vi "Write Maximum Channel Length.vi"(8 "error in (no error)":errorcluster, 10 "maximum data length":i32, 11 "Data in":refnum<class "Data.lvclass">) -> (0 "error out":errorcluster, 3 "Data out":refnum<class "Data.lvclass">)   [LabVIEW 2017, in "Data.lvclass"]
uses:
  <vilib>/addons/_NISVFA/_Shared subVIs/Data Objects/Data/Data.lvclass
  <vilib>/addons/_NISVFA/_Shared subVIs/Data Objects/Data/Data.lvclass/Data.ctl
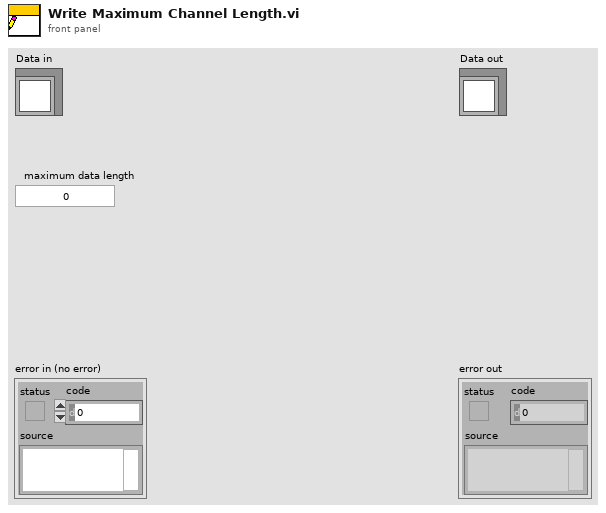
[diagram p1: front panel]
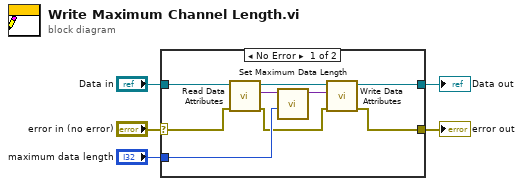
[diagram p0: block diagram]
diagram:
  n1 = case shown="No Error" "error in (no error)" {
    selector: "error in (no error)" -> [w7 w15]
    tunnel: [w6 w15] -> w4
    tunnel: [w13 w16] -> w2
    tunnel: "Data in" -> [w14 w16]
    tunnel: "maximum data length" -> [w10 _]
    frame No Error {
      n2 = call <vilib>:"Read Data Attributes.vi"("error in (no error)"=w7, "Data in"=w14) -> ("error out"=w8:errorcluster, "data attributes"=w12:variant, "Data out"=w9:refnum<class "Data.lvclass">)  [unwired: 7 in]
      n3 = call <vilib>:"Set Maximum Data Length.vi"("maximum data length"=w10, "variant in"=w12) -> ("variant out"=w11:variant)  [unwired: 9 in]
      n4 = call <vilib>:"Write Data Attributes.vi"("error in (no error)"=w8, "data attributes"=w11, "Data in"=w9) -> ("error out"=w6:errorcluster, "Data out"=w13:refnum<class "Data.lvclass">)  [unwired: 7 in]
    }
    frame Error {
    }
  }
  "error out" <- w4
  "Data out" <- w2
